vi "CreateFilenameByTimeStamp.vi"(9 "error in (no error)":errorcluster) -> (2 "Filename":string, 6 "error out":errorcluster)   [LabVIEW 2009]
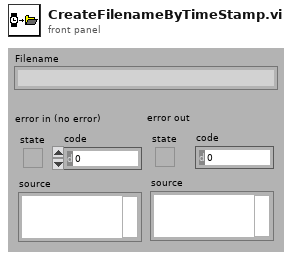
[diagram p1: front panel]
types:
  T1 = cluster{"second":i32, "minute":i32, "hour":i32, "day of month":i32, "month":i32, "year":i32, "day of week":i32, "day of year":i32, "is DST":i32}
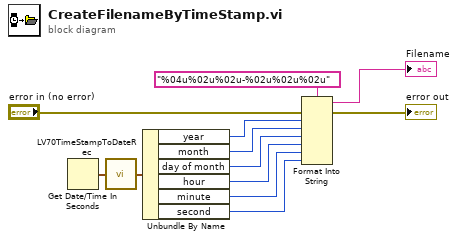
[diagram p0: block diagram]
diagram:
  n1 = Get Date/Time In Seconds() -> (seconds since 1Jan1904=w2:timestamp)
  n2 = call <vilib>:"LV70TimeStampToDateRec.vi"("time stamp"=w2) -> ("date time rec"=w3:T1)
  n3 = Unbundle By Name(w3) -> ("year"=w4:i32, "month"=w5:i32, "day of month"=w6:i32, "hour"=w7:i32, "minute"=w8:i32, "second"=w9:i32)
  n4 = Format Into String(format string="%04u%02u%02u-%02u%02u%02u" ("chaîne de format"), error in="error in (no error)", w4, w5, w6, w7, w8, w9) -> (resulting string=→"Filename":string, error out=→"error out":errorcluster)  [unwired: 1 in]
